vi "Read Analogue.vi"(8 "error in (no error)":errorcluster, 11 "KE27XX DMM in":refnum<class "Keithley 27XX DMM.lvclass">) -> (0 "error out":errorcluster, 2 "Waveforms":waveform(dbl)[](array[waveform]), 3 "KE27XX DMM out":refnum<class "Keithley 27XX DMM.lvclass">)   [LabVIEW 2025, in "DMM.lvlib" / "Keithley 27XX DMM.lvclass"]
uses:
  Keithley 27XX DMM.lvclass
  C:/Users/Public/Documents/Sandia National Labs/TSS Plugin/Abstract Engine.lvlibp/Abstract Instrument/Abstract Instrument.lvclass
  Keithley 27XX DMM.lvclass/Keithley 27XX DMM.ctl
  <instrlib>/Keithley 27XX/Keithley 27XX.lvlib
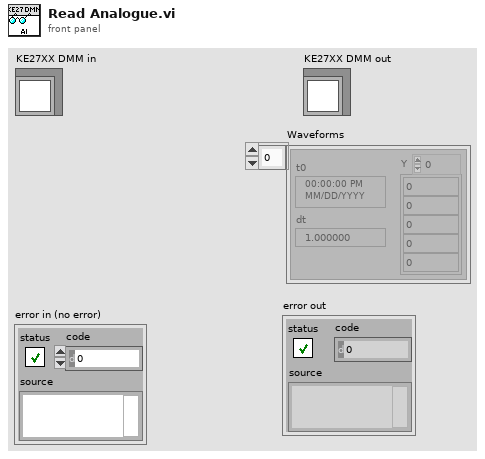
[diagram p1: front panel]
types:
  T1 = typedef "Abstract Engine.lvlibp/Abstract Instrument.lvclass/Channel.ctl" = cluster{"Alias":string, "DataType":enum16{"Anaolg Input", "Waveform"}, "Unit":enum16{"---", "V", "A", "Ohm", "Hz", "uF", "degC", "deg"}, "Upper limit":dbl, "Lower limit":dbl, "Measurement":variant}
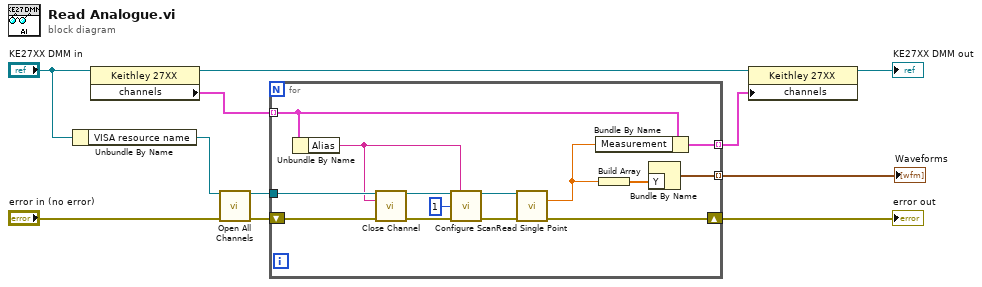
[diagram p0: block diagram]
diagram:
  n1 = Unbundle By Name("KE27XX DMM in") -> ("VISA resource name"=w9:refnum<visa-resource-name>)
  n2 = property class="Keithley 27XX"(reference="KE27XX DMM in") -> (reference out=w5:refnum<class "Keithley 27XX DMM.lvclass">, "channels"=w3:T1[])  [unwired: 1 in, 1 out]
  n3 = call <instrlib>:"Open All Channels.vi"("VISA resource name"=w9, "error in (no error)"="error in (no error)") -> ("VISA resource name out"=w8:refnum<visa-resource-name>, "error out"=w7:errorcluster)  [unwired: 12 in]
  n4 = for {
    tunnel: w8 -> [w25]
    shift-right: [w18] -> w6
    shift-left: w7 -> [w24]
    tunnel: w3 -> [w16] mode=indexing
    tunnel: [w15] -> w2 mode=indexing
    tunnel: [w12] -> w1 mode=indexing
    n5 = Unbundle By Name(w16) -> ("Alias"=w17:string)
    n6 = call <instrlib>:"Close Channel.vi"("VISA resource name"=w25, "Channel List (101)"=w17, "error in (no error)"=w24) -> ("VISA resource name out"=w23:refnum<visa-resource-name>, "error out"=w22:errorcluster)  [unwired: 11 in]
    n7 = call <instrlib>:"Configure Scan.vi"("VISA resource name"=w23, "Channel List (101:110)"=w17, "Sample Count (100)"=1, "error in (no error)"=w22) -> ("VISA resource name out"=w20:refnum<visa-resource-name>, "error out"=w19:errorcluster)  [unwired: 10 in]
    n8 = call <instrlib>:"Read Single Point.vi"("VISA resource name"=w20, "error in (no error)"=w19) -> ("Measurement Data"=w14:dbl, "error out"=w18:errorcluster)  [unwired: 11 in, 1 out]
    n9 = Bundle By Name(cluster=w16, "Measurement"=w14) -> (w15:T1)
    n10 = Build Array(w14) -> (w13:dbl[])
    n11 = Bundle By Name("Y"=w13) -> (w12:waveform(dbl))  [unwired: 1 in]
  }
  "error out" <- w6
  "Waveforms" <- w1
  n12 = property class="Keithley 27XX"(reference=w5, "channels"=w2) -> (reference out=→"KE27XX DMM out":refnum<class "Keithley 27XX DMM.lvclass">)  [unwired: 1 in, 1 out]
